vi "sub vi - AI USB4704 (3) v73.vi"(0 "Task0":i32, 5 "Task1":i32, 7 "Task2":i32, 11 "SAMPLES":dbl) -> (4 "data 0":waveform(dbl)[](array[waveform]), 6 "data 1":waveform(dbl)[](array[waveform]), 8 "data 2":waveform(dbl)[](array[waveform]), 10 "loop time":dbl format="%.6g", 15 "error array":errorcluster[](array[cluster]))   [LabVIEW 2017]
uses:
  <userlib>/DAQNavi Polymorphic VI/read/DAQNavi Read (Analog 1D Wfm NChan NSamp).vi
panel:
  in  "Tab Control":enum32{"USB #0", "USB #1", "USB #2"}(tab)
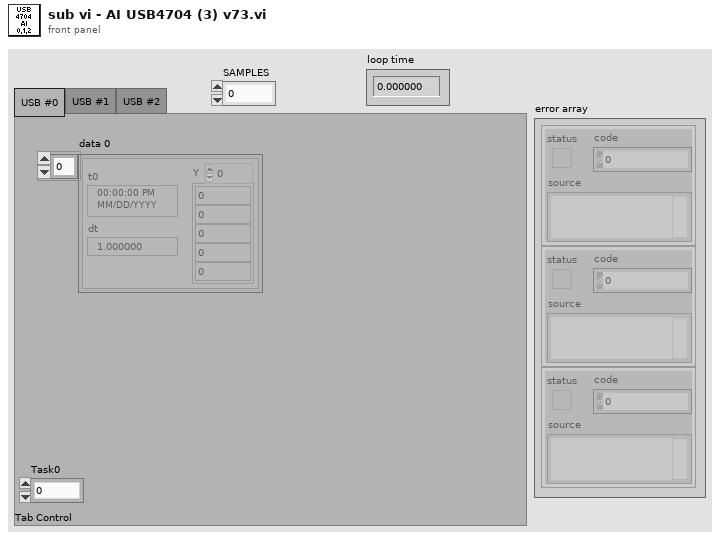
[diagram p1: front panel]
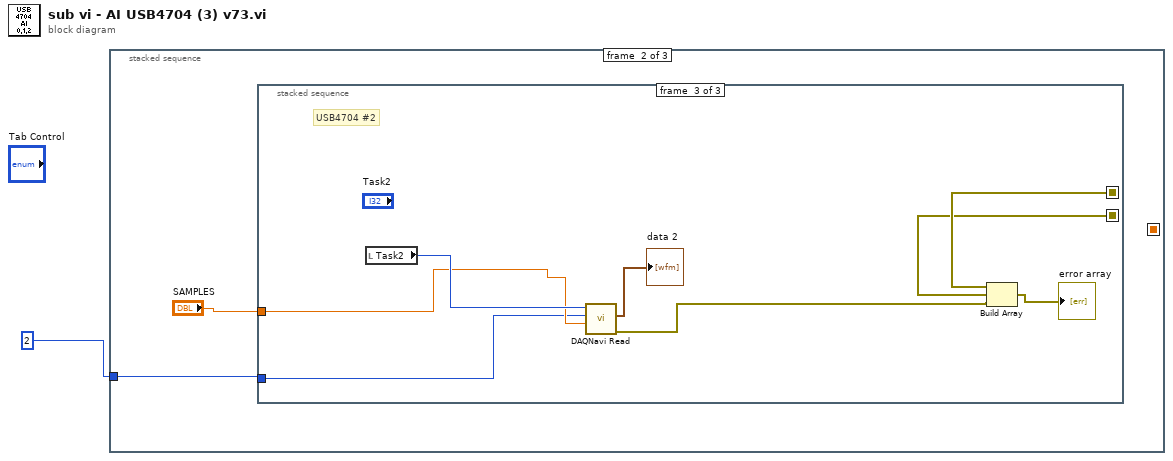
[diagram p0: block diagram]
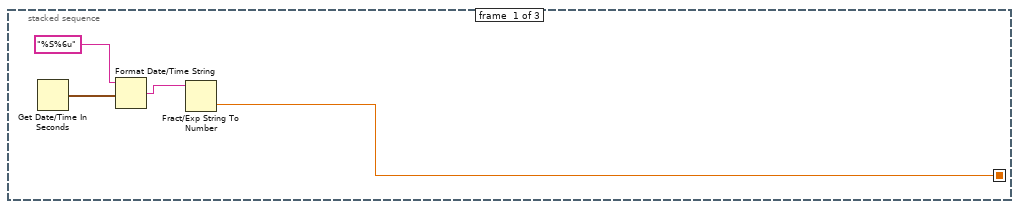
[diagram p2: hidden frame]
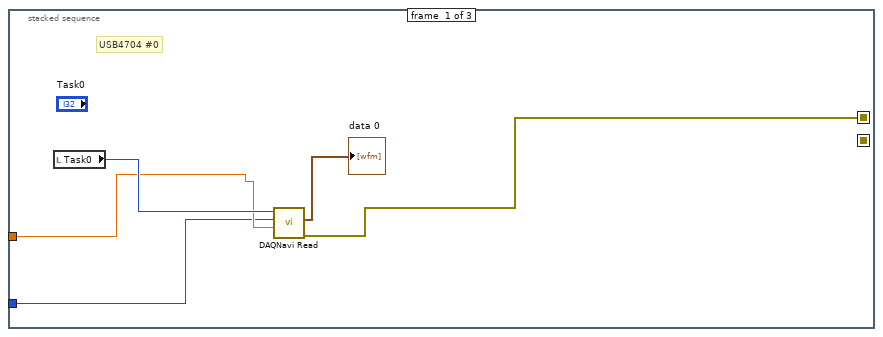
[diagram p3: hidden frame]
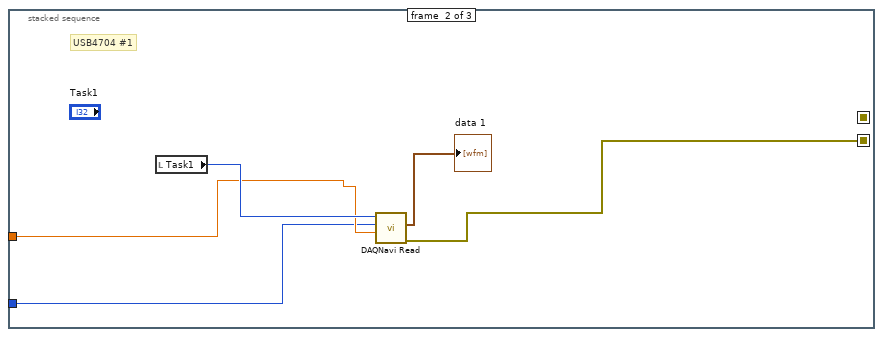
[diagram p4: hidden frame]
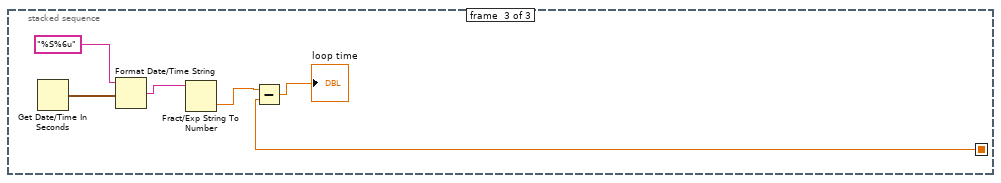
[diagram p5: hidden frame]
diagram:
  n1 = stacked-sequence {
    seq-local: [w2 _ _] -> [_ _ w27]
    tunnel: 2 -> [_ w7 _]
    frame #0 {
      n2 = Get Date/Time In Seconds() -> (seconds since 1Jan1904=w4:timestamp)
      n3 = Format Date/Time String(time format string (%c)="%S%6u", seconds (now)=w4) -> (date/time string=w3:string)  [unwired: 1 in]
      n4 = Fract/Exp String To Number(string=w3) -> (number=w2:dbl)  [unwired: 3 in, 1 out]
    }
    frame #1 {
      n5 = stacked-sequence {
        seq-local: [w10 _ _] -> [_ _ w22]
        seq-local: [_ w16 _] -> [_ _ w21]
        tunnel: "SAMPLES" -> [w11 w15 w24]
        tunnel: w7 -> [w9 w14 w19]
        frame #0 {
          # "USB4704 #0"
          n6 = local read "Task0"() -> (w12:i32)
          n7 = call-poly <userlib>:"DAQNavi Read.vi"("number of samples per channel to read"=w11, "timeout"=w9, "task in"=w12) -> ("error out"=w10:errorcluster, "data"=→"data 0":waveform(dbl)[])  [unwired: 1 in, 6 out]
        }
        frame #1 {
          # "USB4704 #1"
          n8 = local read "Task1"() -> (w17:i32)
          n9 = call-poly <userlib>:"DAQNavi Read.vi"("number of samples per channel to read"=w15, "timeout"=w14, "task in"=w17) -> ("error out"=w16:errorcluster, "data"=→"data 1":waveform(dbl)[])  [unwired: 1 in, 6 out]
        }
        frame #2 {
          # "USB4704 #2"
          n10 = local read "Task2"() -> (w25:i32)
          n11 = call-poly <userlib>:"DAQNavi Read.vi"("number of samples per channel to read"=w24, "timeout"=w19, "task in"=w25) -> ("error out"=w23:errorcluster, "data"=→"data 2":waveform(dbl)[])  [unwired: 1 in, 6 out]
          n12 = Build Array(w22, w21, w23) -> (→"error array":errorcluster[])
        }
      }
    }
    frame #2 {
      n13 = Get Date/Time In Seconds() -> (seconds since 1Jan1904=w30:timestamp)
      n14 = Format Date/Time String(time format string (%c)="%S%6u", seconds (now)=w30) -> (date/time string=w29:string)  [unwired: 1 in]
      n15 = Fract/Exp String To Number(string=w29) -> (number=w28:dbl)  [unwired: 3 in, 1 out]
      n16 = Subtract(x=w28, y=w27) -> (x-y=→"loop time":dbl)
    }
  }
